vi "svm_predict.vi"(8 "error in (no error)":errorcluster, 10 "X":T1[](array[typedef])=[{"index"=0, "value"=0.0}], 11 "Model":T2) -> (0 "error out":errorcluster, 3 "Predicted label":dbl)   [LabVIEW 2014]
doc: "This function does classification or regression on a test vector x given a model.\n\nFor a classification model, the predicted class for x is returned.\nFor a regression model, the function value of x calculated using the model is returned. For an one-class model, +1 or -1 is returned."
uses:
  Controls/svm_model.ctl
  Controls/svm_parameter.ctl
  Controls/svm_type.ctl
  Controls/svm_kernel_type.ctl
  Controls/svm_node.ctl
  <vilib>/oysstu/LVLibSVM/bin/x64/LVLibSVM.dll
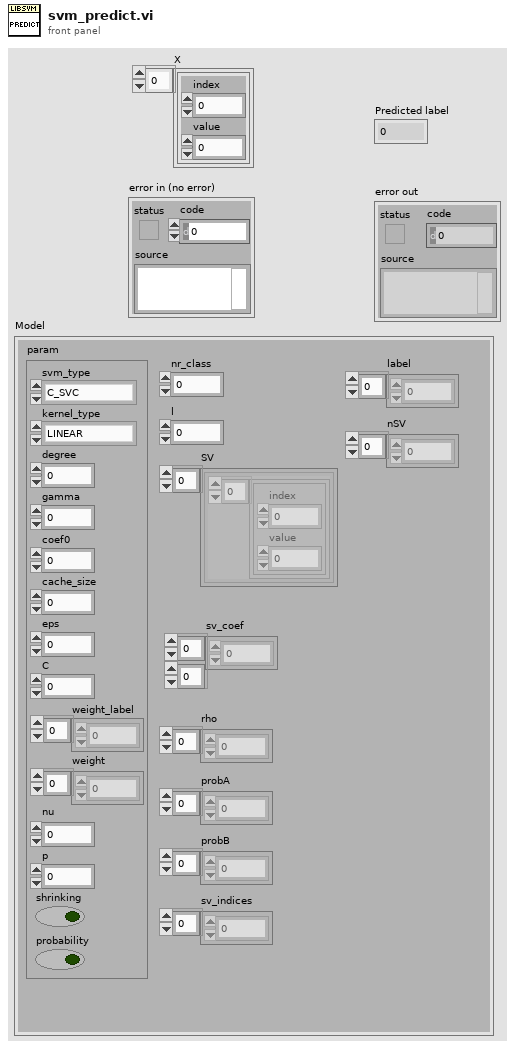
[diagram p1: front panel]
types:
  T1 = typedef "svm_node.ctl" = cluster{"index":i32, "value":dbl}
  T2 = typedef "svm_model.ctl" = cluster{"param":T3, "nr_class":i32, "l":i32, "SV":cluster{"Array":T1[]}[], "sv_coef":dbl[][], "rho":dbl[], "probA":dbl[], "probB":dbl[], "sv_indices":i32[], "label":i32[], "nSV":i32[]}
  T3 = typedef "svm_parameter.ctl" = cluster{"svm_type":T4, "kernel_type":T5, "degree":i32, "gamma":dbl, "coef0":dbl, "cache_size":dbl, "eps":dbl, "C":dbl, "weight_label":i32[], "weight":dbl[], "nu":dbl, "p":dbl, "shrinking":bool, "probability":bool}
  T4 = typedef "svm_type.ctl" = enum32{"C_SVC", "NU_SVC", "ONE_CLASS", "EPSILON_SVR", "NU_SVR"}
  T5 = typedef "svm_kernel_type.ctl" = enum32{"LINEAR", "POLY", "RBF", "SIGMOID", "PRECOMPUTED"}
  T6 = typedef "svm_node_padded.ctl" = cluster{"index":i32, "padding":i32, "value":dbl}
  T7 = typedef "svm_model_padded.ctl" = cluster{"param":T3, "nr_class":i32, "l":i32, "SV":cluster{"Array":T6[]}[], "sv_coef":dbl[][], "rho":dbl[], "probA":dbl[], "probB":dbl[], "sv_indices":i32[], "label":i32[], "nSV":i32[]}
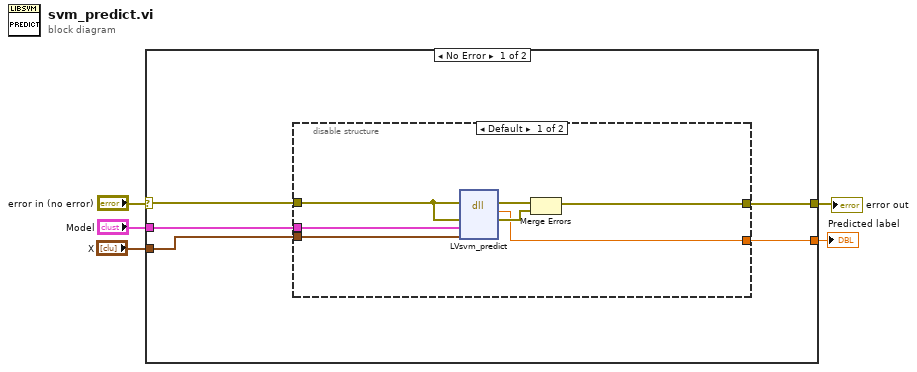
[diagram p0: block diagram]
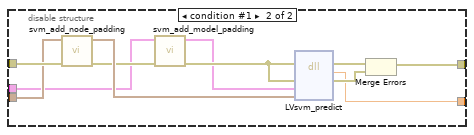
[diagram p2: hidden frame]
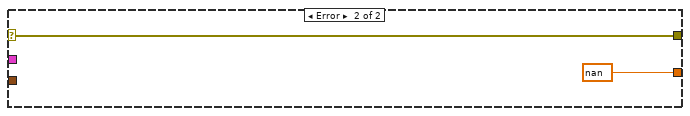
[diagram p3: hidden frame]
diagram:
  n1 = case shown="No Error" "error in (no error)" {
    selector: "error in (no error)" -> [w10 w30]
    tunnel: [w9 w30] -> w5
    tunnel: "Model" -> [w8 _]
    tunnel: "X" -> [w7 _]
    tunnel: [w6 nan ("predicted label")] -> w1
    frame No Error {
      n2 = disable-structure shown="Default" {
        disable-tunnel: w10 -> [w17 w24]
        disable-tunnel: [w14 w26] -> w9
        disable-tunnel: w8 -> [w13 w19]
        disable-tunnel: w7 -> [w12 w23]
        disable-tunnel: [w11 w25] -> w6
        frame condition #0 (active) {
          n3 = dll-call lib="C:/Program Files/National Instruments/LabVIEW 2014/vi.lib/oysstu/LVLibSVM/bin/x64/LVLibSVM.dll" fn="LVsvm_predict"(error in=w17, "lvErr"=w17, "model_in"=w13, "x_in"=w12) -> (error out=w16:errorcluster, "predicted label"=w11:dbl, "lvErr"=w15:errorcluster)  [unwired: 4 in, 1 out]
          n4 = Merge Errors(w16, w15) -> (w14:errorcluster)
        }
        frame condition #1 {
          n5 = call "svm_add_node_padding.vi"("error in (no error)"=w24, "Nodes"=w23) -> ("error out"=w21:errorcluster, "Padded nodes"=w22:T6[])  [unwired: 8 in]
          n6 = call "svm_add_model_padding.vi"("error in (no error)"=w21, "Model"=w19) -> ("error out"=w20:errorcluster, "Padded model"=w18:T7)  [unwired: 8 in]
          n7 = dll-call lib="C:/Program Files/National Instruments/LabVIEW 2014/vi.lib/oysstu/LVLibSVM/bin/x64/LVLibSVM.dll" fn="LVsvm_predict"(error in=w20, "lvErr"=w20, "model_in"=w18, "x_in"=w22) -> (error out=w28:errorcluster, "predicted label"=w25:dbl, "lvErr"=w27:errorcluster)  [unwired: 4 in, 1 out]
          n8 = Merge Errors(w28, w27) -> (w26:errorcluster)
        }
      }
    }
    frame Error {
    }
  }
  "error out" <- w5
  "Predicted label" <- w1
